vi "extScanStepLogic.vi"() -> (3 "timedOut":bool)   [LabVIEW 2014]
uses:
  <vilib>/Platform/TimedLoop/XDataNode/timing_clust.ctl
  <vilib>/Platform/TimedLoop/XDataNode/nitl_modes.ctl
  <vilib>/Platform/TimedLoop/XDataNode/wakeup.ctl
  extScanGlobalVars.vi
  <vilib>/rvi/Emulation/niFpgaSctlEmulationGetInTimedLoop.vi
  <vilib>/rvi/Emulation/niFpgaEmulationReportErrorSimple.vi
  <vilib>/rvi/Emulation/niFpgaGetClockAttributes.vi
  <vilib>/rvi/Emulation/niFpgaCriticalErrorInLSC.vi
  Sequencer/sequencerGlobVars.vi
  <vilib>/Platform/TimedLoop/XDataNode/XDataNode.xnode
  <vilib>/Platform/TimedLoop/XDataNode/XDNodeRunTimeDep.lvlib
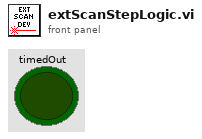
[diagram p1: front panel]
types:
  T1 = typedef "XDNodeRunTimeDep.lvlib/timing_clust.ctl" = cluster{"Expected End [f-1]":u64, "Actual End [f-1]":u64, "Finished Late? [f-1]":bool, "Expected End [i-1]":u64, "Actual End [i-1]":u64, "Finished Late? [i-1]":bool, "Expected Start [i]":u64, "Actual Start [i]":u64, "Expected Start [f]":u64, "Actual Start [f]":u64, "Source Name":string, "Structure Name":string, "Period":i64, "Deadline":i64, "Offset":i64, "Start":i64, "Priority":i32, "Timeout":i32, "Mode":T2, "Wakeup Reason":T3, "Error":errorcluster, "Source Type":string, "Secondary Source Type":string, "Global End Time":u64, "Global Start Time":u64, "Frame Duration":u64, "Iteration Duration":u64, "Assigned CPU":i32, "I/O Scan Engine Mode":u32}
  T2 = typedef "XDNodeRunTimeDep.lvlib/nitl_modes.ctl" = enum32{"No Change", "Process missed periods, maintain original phase", "Discard missed periods, maintain original phase", "Process missed periods, ignore original phase", "Discard missed periods, ignore original phase"}
  T3 = typedef "XDNodeRunTimeDep.lvlib/wakeup.ctl" = enum32{"Normal", "Aborted", "Asynchronous wakeup", "Timing source error", "Timed loop error", "Timeout"}
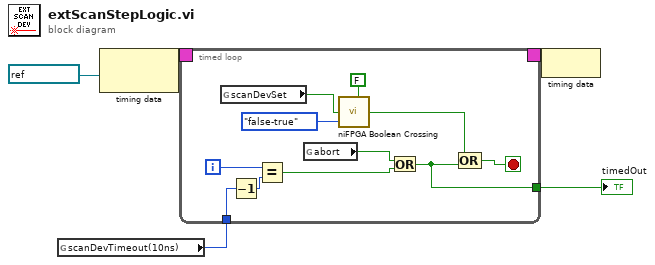
[diagram p0: block diagram]
diagram:
  n1 = global read "extScanGlobalVars.vi" "scanDevTimeout(10ns)"() -> (w2:i32)
  n2 = node-c288(refnum<k21> "100MHz" ("FPGA Clock")) -> (w5:T1)
  n3 = timed-loop {
    timing: w5 -> [_]
    timing-out: [_] -> w4
    tunnel: w2 -> [w13]
    tunnel: [w8] -> w1
    i -> [w6]
    stop <- w12 stop-if-true
    n4 = global read "extScanGlobalVars.vi" "scanDevSet"() -> (w15:bool)
    n5 = Decrement(x=w13) -> (x-1=w7:i32)
    n6 = Equal?(x=w6, y=w7) -> (x = y?=w9:bool)
    n7 = global read "sequencerGlobVars.vi" "abort"() -> (w10:bool)
    n8 = call <vilib>:"niFPGA Boolean Crossing.vi"("input"=w15, "direction"=enum8{"either", "false-true", "true-false"}."false-true", "initialize"=FALSE) -> ("crossing"=w11:bool)  [unwired: 6 in]
    n9 = Or(x=w10, y=w9) -> (x .or. y?=w8:bool)
    n10 = Compound Arithmetic op=OR(w11, w8) -> (w12:bool)
  }
  "timedOut" <- w1
  n11 = node-c288(w4) -> ()
